vi "8-State of Plane.vi"() -> ()   [LabVIEW 2020]
panel:
  out "Time Elapsed(h)":i32
  out "Arrived in Destination Point":bool
  out "State of Plane (Indicator)":T1={"Departure Point"="Moscow", "Arrival Point"="New York", "Number of Passengers "=300.0, "Crew on board"="1xPilot\n2xCo-Pilot\n10xCabin Personnel", "Course(Degrees)"=187.6, "Acceleration (nm/h2)"=50.0, "Velocity (kts)"=0.0, "Longitude"=265611.0, "Latitude"=146310.0, "Destination Latitude"=146310.0, "Destination Longitude"=265611.0} {"Destination Longitude" format="%<%Hº%M'%S\"%u>t"; "Destination Latitude" format="%<%Hº%M'%S\"%u>t"; "Latitude" format="%<%Hº%M'%S\"%u>t"; "Longitude" format="%<%Hº%M'%S\"%u>t"}
  in  "Auto-pilot Error Range(%)":dbl=1.0
  in  "State of Plane (Control)":T2={"Departure Point"="Moscow", "Arrival Point"="New York", "Number of Passengers "=300.0, "Crew on board"="1xPilot\n2xCo-Pilot\n10xCabin Personnel", "Course(Degrees)"=187.53, "Acceleration (nm/h2)"=50.0, "Initial Velocity (kts)"=0.0, "Longitude"=136446.0, "Latitude"=199460.0, "Destination Latitude"=146310.0, "Destination Longitude"=-265610.0} {"Destination Longitude" format="%<%Hº%M'%S\"%u>t"; "Destination Latitude" format="%<%Hº%M'%S\"%u>t"; "Latitude" format="%<%Hº%M'%S\"%u>t"; "Longitude" format="%<%Hº%M'%S\"%u>t"; "Course(Degrees)" format="%#_8g"}
  # "Min error is %1 for this \"Course\". If it is set less than 1%, \ndestination point may be missed and program may not halt.\nUser can set more accurate  \"Course\" or alter it while on the \nfly in order to adjust the land-off point. Error can be selected\n higher for the program to halt properly if the \"Course\" is roughly\n calculated."
  # "Course is set according to trigonometric unit  circle, NOT\nto geographical compass.(there is 90 deg phase shift)"
  # "kts(knots) ; nm(nautical mile) ;  h(hours)"
  # "[V]= kts(knots)  ;   1kts = 1nm/h\n\n1º = 60'  ;   1' = 60\"\n\n1' = 1nm = 1852m"
  # "Position of Moscow     55º24'20\" N\nAirport                            37º54'06\" E\n\nPosition of New York   40º38'30\" N\nAirport                            73º46'51\" W"
  # "The direct course should be set as 187.6 in order to arrive\nNew York from Moscow."
  # "\"N\" and \"E\" directions are assumed as positive. \"W\" and \n\"S\" as negative."
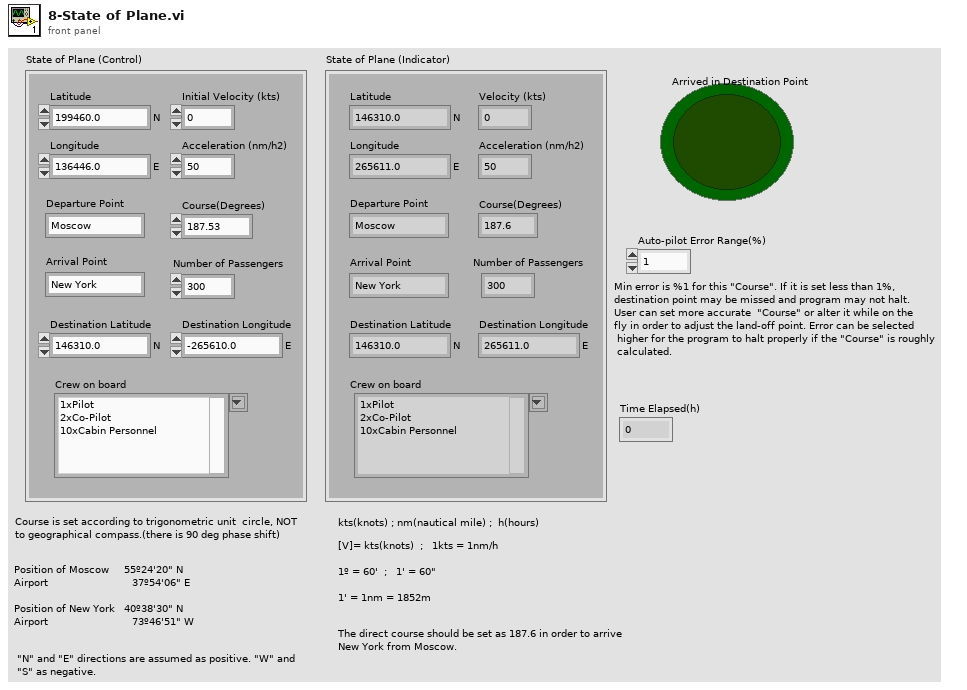
[diagram p1: front panel]
types:
  T1 = cluster{"Departure Point":string, "Arrival Point":string, "Number of Passengers ":dbl, "Crew on board":string, "Course(Degrees)":dbl, "Acceleration (nm/h2)":dbl, "Velocity (kts)":dbl, "Longitude":dbl, "Latitude":dbl, "Destination Latitude":dbl, "Destination Longitude":dbl}
  T2 = cluster{"Departure Point":string, "Arrival Point":string, "Number of Passengers ":dbl, "Crew on board":string, "Course(Degrees)":dbl, "Acceleration (nm/h2)":dbl, "Initial Velocity (kts)":dbl, "Longitude":dbl, "Latitude":dbl, "Destination Latitude":dbl, "Destination Longitude":dbl}
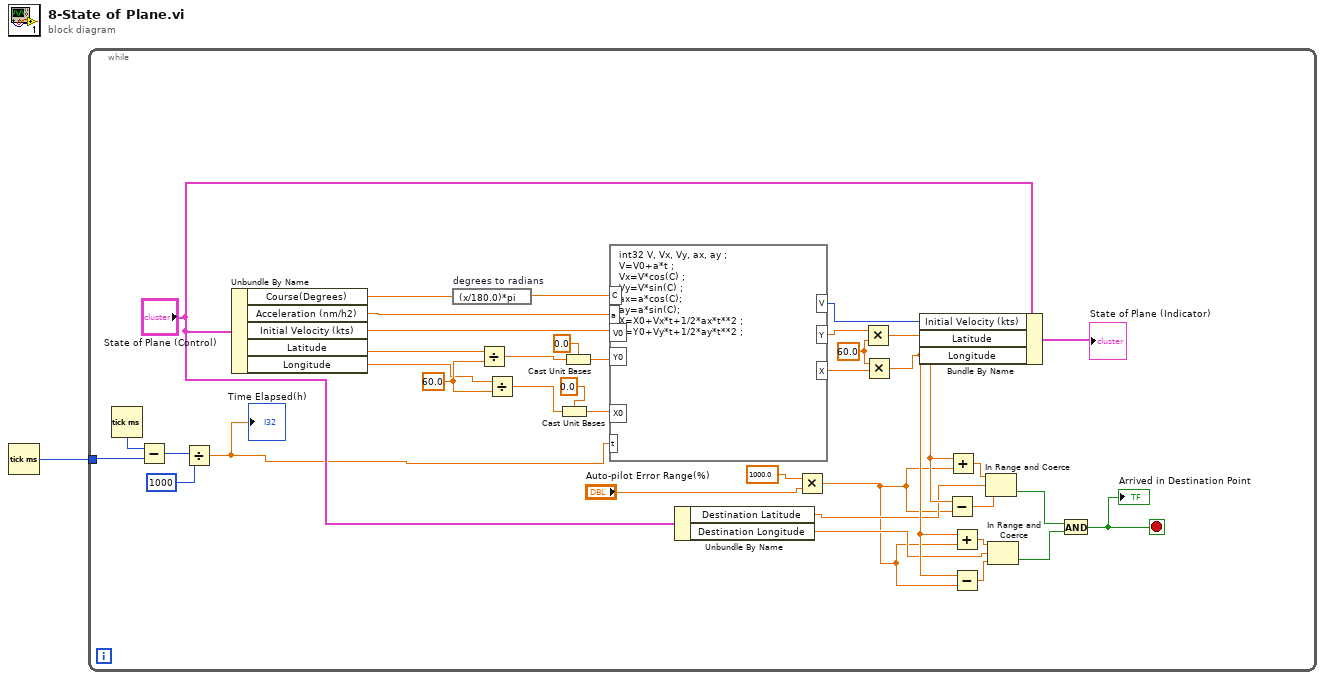
[diagram p0: block diagram]
diagram:
  n1 = Tick Count (ms)() -> (millisecond timer value=w1:u32)
  n2 = while {
    tunnel: w1 -> [w30]
    stop <- w3 stop-if-true
    w27 = 60.0
    w36 = 60.0
    n3 = Tick Count (ms)() -> (millisecond timer value=w31:u32)
    n4 = Subtract(x=w31, y=w30) -> (x-y=w29:u32)
    n5 = Divide(x=w29, y=u32 1000) -> (x/y=w2:dbl)
    "Time Elapsed(h)" <- w2
    n6 = Unbundle By Name("State of Plane (Control)") -> ("Course(Degrees)"=w26:dbl, "Acceleration (nm/h2)"=w39:dbl, "Initial Velocity (kts)"=w24:dbl, "Latitude"=w35:dbl, "Longitude"=w34:dbl)
    n7 = expression code="(x/180.0)*pi" "degrees to radians"(w26) -> (w25:dbl)
    n8 = Divide(x=w35, y=w36) -> (x/y=w33:dbl)
    n9 = Divide(x=w34, y=w36) -> (x/y=w32:dbl)
    n10 = Cast Unit Bases(0:w32, 1:0.0 ("unit (none)")) -> (2:w8:dbl)
    n11 = Cast Unit Bases(0:w33, 1:0.0 ("unit (none)")) -> (2:w9:dbl)
    n12 = formula code="int32 V, Vx, Vy, ax, ay ;\nV=V0+a*t ;\nVx=V*cos(C) ;\nVy=V*sin(C) ;\nax=a*cos(C);\nay=a*sin(C);\nX=X0+Vx*t+1/2*ax*t**2 ;\nY=Y0+Vy*t+1/2*ay*t**2 ;"("a"=w39, "C"=w25, "X0"=w8, "Y0"=w9, "V0"=w24, "t"=w2) -> ("X"=w10:dbl, "Y"=w11:dbl, "V"=w23:i32)
    n13 = Unbundle By Name("State of Plane (Control)") -> ("Destination Latitude"=w13:dbl, "Destination Longitude"=w12:dbl)
    n14 = Multiply(x=1000.0, y="Auto-pilot Error Range(%)") -> (x*y=w4:dbl)
    n15 = Multiply(x=w11, y=w27) -> (x*y=w15:dbl)
    n16 = Multiply(x=w27, y=w10) -> (x*y=w14:dbl)
    n17 = Bundle By Name(cluster="State of Plane (Control)", "Initial Velocity (kts)"=w23, "Latitude"=w15, "Longitude"=w14) -> (→"State of Plane (Indicator)":T2)
    n18 = Subtract(x=w15, y=w4) -> (x-y=w17:dbl)
    n19 = Add(x=w15, y=w4) -> (x+y=w20:dbl)
    n20 = Add(x=w14, y=w4) -> (x+y=w18:dbl)
    n21 = Subtract(x=w14, y=w4) -> (x-y=w19:dbl)
    n22 = In Range and Coerce(upper limit=w20, x=w13, lower limit=w17) -> (In Range?=w22:bool)  [unwired: 1 out]
    n23 = In Range and Coerce(upper limit=w18, x=w12, lower limit=w19) -> (In Range?=w21:bool)  [unwired: 1 out]
    n24 = And(x=w22, y=w21) -> (x .and. y?=w3:bool)
    "Arrived in Destination Point" <- w3
  }
